vi "DB_Insert.vi"() -> ()   [LabVIEW 2020]
uses:
  <vilib>/addons/database/Connection.llb/DB Tools Open Connec (String).vi
  <vilib>/addons/database/_DB Variant To Data/Database Variant To Data.xnode
  <vilib>/addons/database/NI_Database_API.lvlib
panel:
  out "Table_ID":string[][](array[string])
  in  "Database":T1(array[cluster])=[{"Nom"="Dupont", "Prénom"="Marie", "age"=32.0, "Sexe"="F", "Métier"="Ingénieure", "Rémunération"=45000.0}, {"Nom"="Dupont", "Prénom"="Jacques", "age"=45.0, "Sexe"="H", "Métier"="Développeur", "Rémunération"=50000.0}, {"Nom"="Leroy", "Prénom"="Sophie", "age"=28.0, "Sexe"="F", "Métier"="Analyste", "Rémunération"=42000.0}, {"Nom"="Bernard", "Prénom"="Thomas", "age"=39.0, "Sexe"="H", "Métier"="Consultant", "Rémunération"=55000.0}, {"Nom"="Moreau", "Prénom"="Claire", "age"=31.0, "Sexe"="F", "Métier"="Designer", "Rémunération"=40000.0}] {"Rémunération" format="%#_g €"}
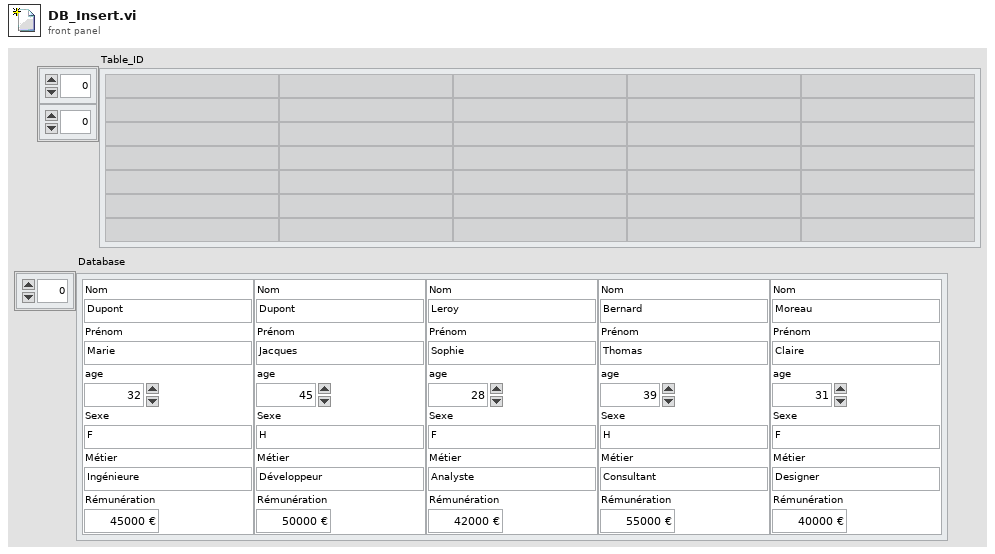
[diagram p1: front panel]
types:
  T1 = cluster{"Nom":string, "Prénom":string, "age":sgl, "Sexe":string, "Métier":string, "Rémunération":sgl}[]
  T2 = typedef "NI_Database_API.lvlib/Conn ObjectReference.ctl" = refnum<k1>
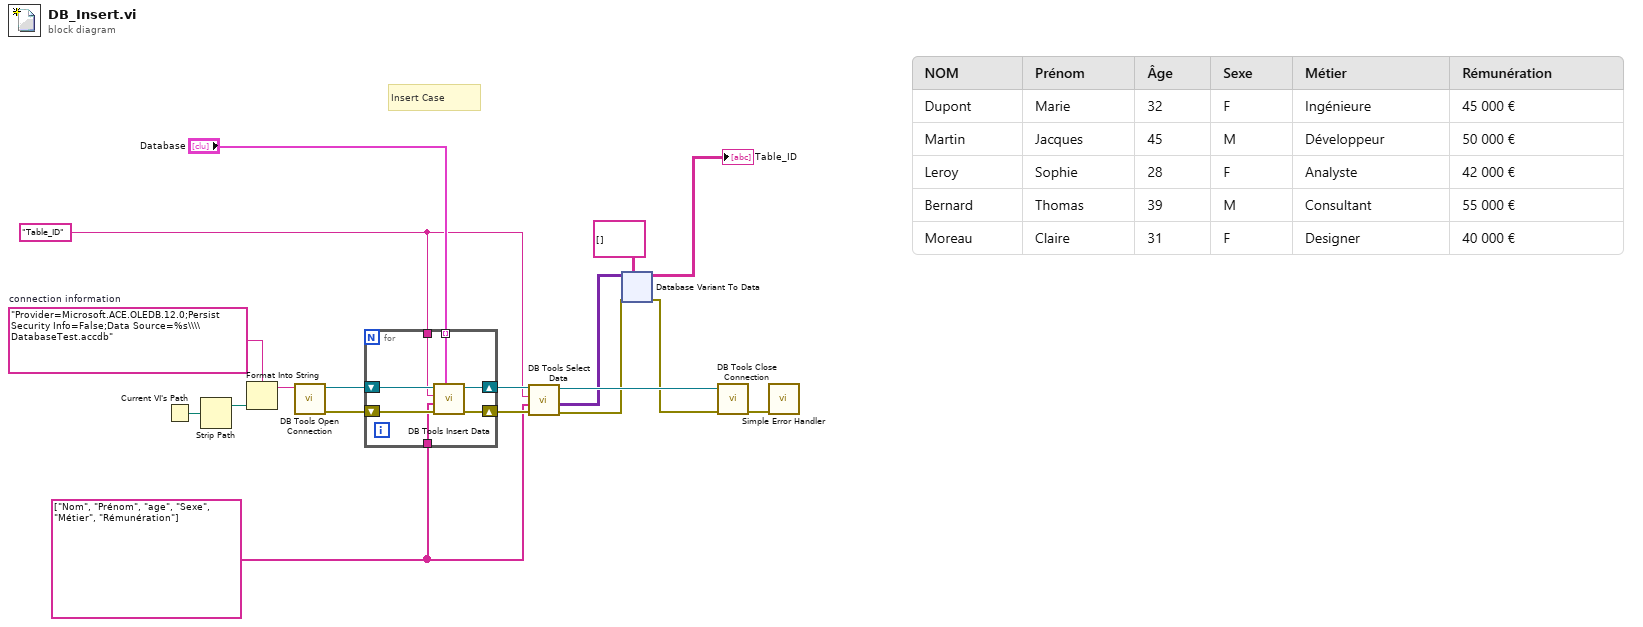
[diagram p0: block diagram]
diagram:
  w6 = string[] ["Nom", "Prénom", "age", "Sexe", "Métier", "Rémunération"] ("columns")
  w7 = "Table_ID" ("table")
  w14 = "Provider=Microsoft.ACE.OLEDB.12.0;Persist Security Info=False;Data Source=%s\\\\DatabaseTest.accdb"  # connection information
  # "Insert Case"
  n1 = Current VI's Path() -> (path=w18:path)
  n2 = Strip Path(path=w18) -> (stripped path=w15:path)  [unwired: 1 out]
  n3 = Format Into String(format string=w14, w15) -> (resulting string=w16:string)  [unwired: 2 in, 1 out]
  n4 = call-poly <vilib>:"DB Tools Open Connection.vi"("connection information"=w16) -> ("error out"=w13:errorcluster, "connection reference"=w12:T2)  [unwired: 7 in]
  n5 = for {
    tunnel: "Database" -> [w23] mode=indexing
    tunnel: w7 -> [w20]
    tunnel: w6 -> [w19]
    shift-right: [w21] -> w9
    shift-left: w13 -> [w25]
    shift-right: [w22] -> w10
    shift-left: w12 -> [w24]
    n6 = call <vilib>:"DB Tools Insert Data.vi"("data"=w23, "error in (no error)"=w25, "columns"=w19, "table"=w20, "connection reference"=w24) -> ("error out"=w21:errorcluster, "connection reference out"=w22:T2)  [unwired: 5 in]
  }
  n7 = call <vilib>:"DB Tools Select Data.vi"("error in (no error)"=w9, "columns"=w6, "table"=w7, "connection reference"=w10) -> ("error out"=w4:errorcluster, "data"=w5:variant[][], "connection reference out"=w8:T2)  [unwired: 2 in]
  n8 = xnode "Database Variant To Data"("database variant"=w5, "error in (no error)"=w4, "type"=string[][] []) -> ("data"=→"Table_ID":string[][], "error out"=w3:errorcluster)
  n9 = call <vilib>:"DB Tools Close Connection.vi"("error in (no error)"=w3, "connection reference"=w8) -> ("error out"=w17:errorcluster)  [unwired: 5 in]
  n10 = call <vilib>:"Simple Error Handler.vi"("error in (no error)"=w17) -> ()  [unwired: 4 in, 5 out]
